vi "GetInstVisaHandle.vi"(8 "error in (no error)":errorcluster, 11 "SpecA_ESA in":refnum<class "SpecA_ESA.lvclass">) -> (0 "error out":errorcluster, 2 "VISA resource name out":refnum<visa-resource-name>, 3 "SpecA_ESA out":refnum<class "SpecA_ESA.lvclass">)   [LabVIEW 2014, in "SpecA_ESA.lvclass"]
uses:
  SpecA_ESA.lvclass
  SpecA_ESA.lvclass/SpecA_ESA.ctl
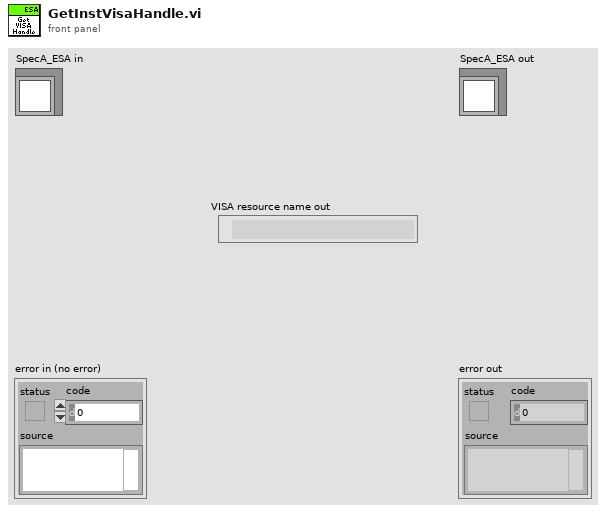
[diagram p1: front panel]
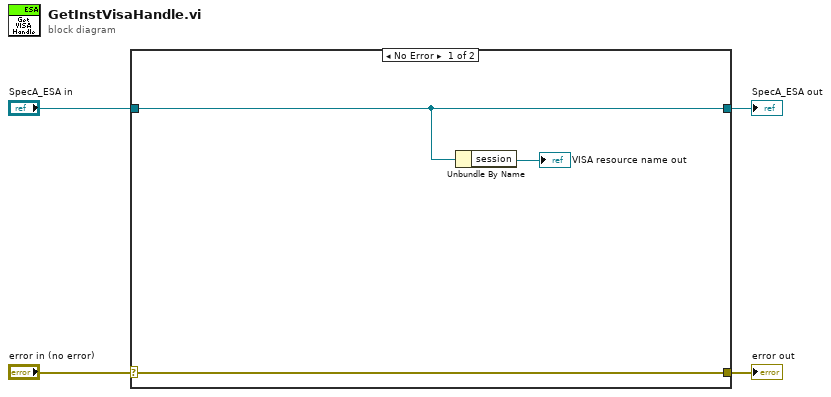
[diagram p0: block diagram]
diagram:
  n1 = case shown="No Error" "error in (no error)" {
    selector: "error in (no error)" -> [w7 w9]
    tunnel: [w7 w9] -> w3
    tunnel: [w6 w8] -> w1
    tunnel: "SpecA_ESA in" -> [w6 w8]
    frame No Error {
      n2 = Unbundle By Name(w6) -> ("session"=→"VISA resource name out":refnum<visa-resource-name>)
    }
    frame Error {
    }
  }
  "error out" <- w3
  "SpecA_ESA out" <- w1
